vi "Moving_detect.vi"(1 "Z":dbl, 2 "Y":dbl, 3 "X":dbl) -> (0 "3轴平方和":dbl)   [LabVIEW 2010]
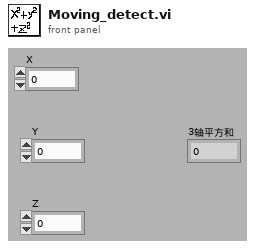
[diagram p1: front panel]
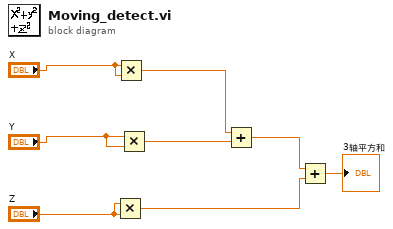
[diagram p0: block diagram]
diagram:
  n1 = Multiply(x="Z", y="Z") -> (x*y=w2:dbl)
  n2 = Multiply(x="X", y="X") -> (x*y=w5:dbl)
  n3 = Multiply(x="Y", y="Y") -> (x*y=w4:dbl)
  n4 = Add(x=w5, y=w4) -> (x+y=w3:dbl)
  n5 = Add(x=w3, y=w2) -> (x+y=→"3轴平方和":dbl)
